vi "Write.vi"(8 "error in (no error)":errorcluster caption="entrée d'erreur (pas d'erreur)", 11 "Class UART Nodon.lvclass En entrée":refnum<class "Class UART Zigbee.lvclass">) -> (0 "error out":errorcluster caption="sortie d'erreur", 3 "Class UART Nodon.lvclass En entrée":refnum<class "Class UART Zigbee.lvclass">)   [LabVIEW 2020, in "Library Instrument & Equipement.lvlib" / "Library UART.lvlib" / "Class UART Zigbee.lvclass"]
uses:
  Class UART Zigbee.lvclass
  C:/Users/ngarcin/OneDrive - Altyor/Standard TB/Class/UART/UART (Default)/Class UART (Default).lvclass
  UART (Default)/Class UART (Default).lvclass
  Class UART Zigbee.lvclass/Class UART Zigbee.ctl
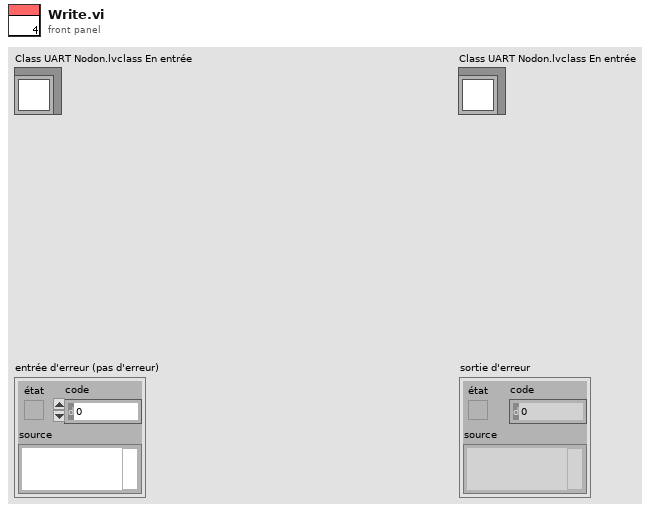
[diagram p1: front panel]
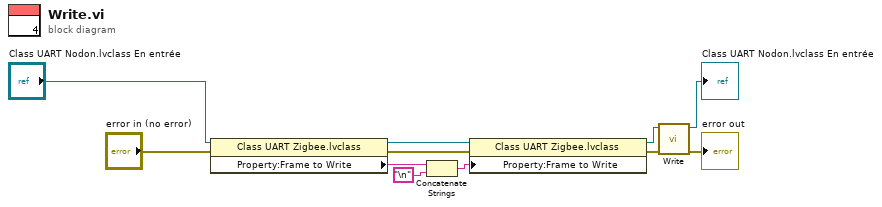
[diagram p0: block diagram]
diagram:
  n1 = property class="Class UART Zigbee.lvclass"(reference="Class UART Nodon.lvclass En entrée", error in="error in (no error)") -> (reference out=w8:refnum<class "Class UART Zigbee.lvclass">, error out=w6:errorcluster, "Property:Frame to Write"=w3:string)
  n2 = Concatenate Strings(w3, "\n") -> (w1:string)
  n3 = property class="Class UART Zigbee.lvclass"(reference=w8, error in=w6, "Property:Frame to Write"=w1) -> (reference out=w4:refnum<class "Class UART Zigbee.lvclass">, error out=w5:errorcluster)
  n4 = call-parent "Write.vi"("error in (no error)"=w5, "Class UART (Default) en entrée"=w4) -> ("error out"=→"error out":errorcluster, "Class UART (Default) en sortie"=→"Class UART Nodon.lvclass En entrée":refnum<class "Class UART Zigbee.lvclass">)  [unwired: 8 in]
